vi "Raw data processing-Ref frame data.vi"(9 "Frame Data in":T5, 11 "Logging queue element":T1={"Imaging Protocol"=enum."Live Imaging", "Number of Trials"=0, "Frame Size"=512, "# Averaged frames"=0, "Dwell time (us)"=0.0, "Index of Z-plane"=0, "Timelapse?"=FALSE, "Logging process is active"=FALSE, "Speed logging enabled"=FALSE, "tdms file ref"=refnum, "path"=path "", "Trial Number"=0, "Expected # points acquired"=FALSE, "Manually stopped"=FALSE, "Last trial"=FALSE, "Ch0 data"=[], "Ch1 data"=[], "Ref Data"=[], "Ref Frame Time"=[], "Image Time"=[], "Continuous Time"=[], "Ref X Length"=0, "Ref Y Length"=0, "# Ref Averaged frames"=0, "Ref Dwell time (us)"=0.0, "Points acquired"={"Ch0 last trial"=0, "Ch1 last trial"=0, "All trials"=0}, "HW Timings File"=refnum} {"Ref Dwell time (us)" format="%#.6g"; "Frame Size" items=["100X100"=100, "128X128"=128, "200X200"=200, "256X256"=256, "512X512"=512, "1024x1024"=1024, "2048x2048"=2048]; "Dwell time (us)" format="%#.6g"}) -> (1 "Frame Data":T5, 2 "Number of points in completed Ref frame":i32, 3 "Ref Frame completed/generate image":bool, 5 "Movement Correction":bool)   [LabVIEW 2017]
uses:
  Typedefs/Frame data dual cluster.ctl
  Typedefs/Logging queue element.ctl
  Typedefs/Imaging Protocols enum.ctl
  Typedefs/Frame Size.ctl
  Typedefs/Acquired points count.ctl
  Global Variables/General Globals.vi
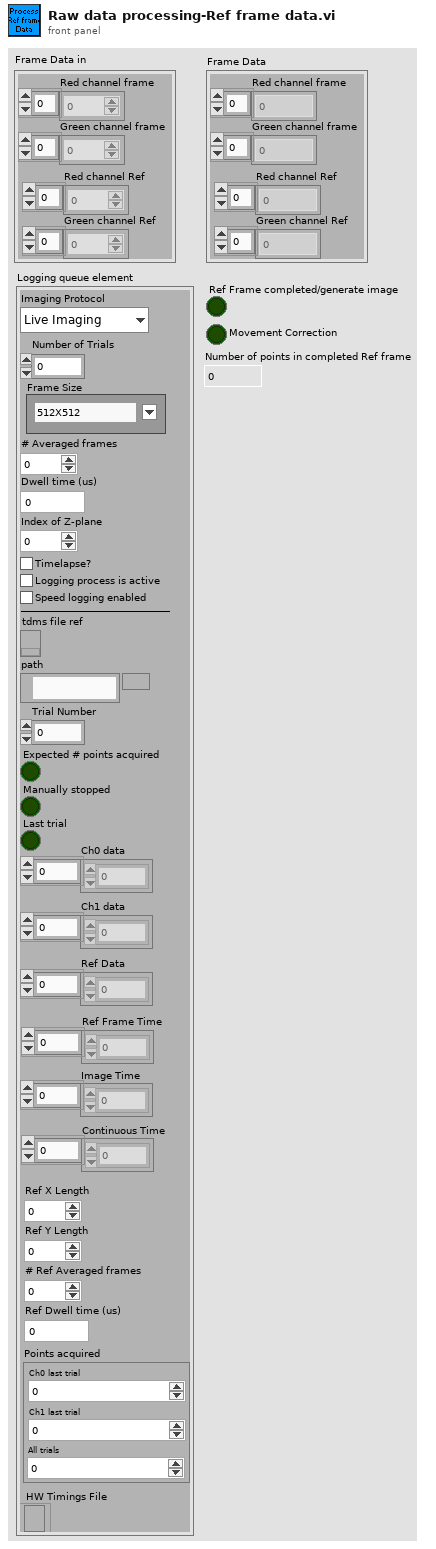
[diagram p1: front panel]
types:
  T1 = typedef "Logging queue element.ctl" = cluster{"Imaging Protocol":T2, "Number of Trials":u16, "Frame Size":T3, "# Averaged frames":u16, "Dwell time (us)":dbl, "Index of Z-plane":i32, "Timelapse?":bool, "Logging process is active":bool, "Speed logging enabled":bool, "tdms file ref":refnum<k34>, "path":path, "Trial Number":i32, "Expected # points acquired":bool, "Manually stopped":bool, "Last trial":bool, "Ch0 data":u32[], "Ch1 data":u32[], "Ref Data":u32[], "Ref Frame Time":u64[], "Image Time":u64[], "Continuous Time":u64[], "Ref X Length":u16, "Ref Y Length":u16, "# Ref Averaged frames":u16, "Ref Dwell time (us)":dbl, "Points acquired":T4, "HW Timings File":refnum<file>}
  T2 = typedef "Imaging Protocols enum.ctl" = enum16{"AOL Z-Stack", "Motor Z Stack", "Functional Acquisition", "Single Plane Acquisition", "Volume Acquisition", "Live Imaging", "Live Plane Imaging", "Live Volume Imaging"}
  T3 = typedef "Frame Size.ctl" = u16
  T4 = typedef "Acquired points count.ctl" = cluster{"Ch0 last trial":u64, "Ch1 last trial":u64, "All trials":u64}
  T5 = typedef "Frame data dual cluster.ctl" = cluster{"Red channel frame":dbl[], "Green channel frame":dbl[], "Red channel Ref":dbl[], "Green channel Ref":dbl[]}
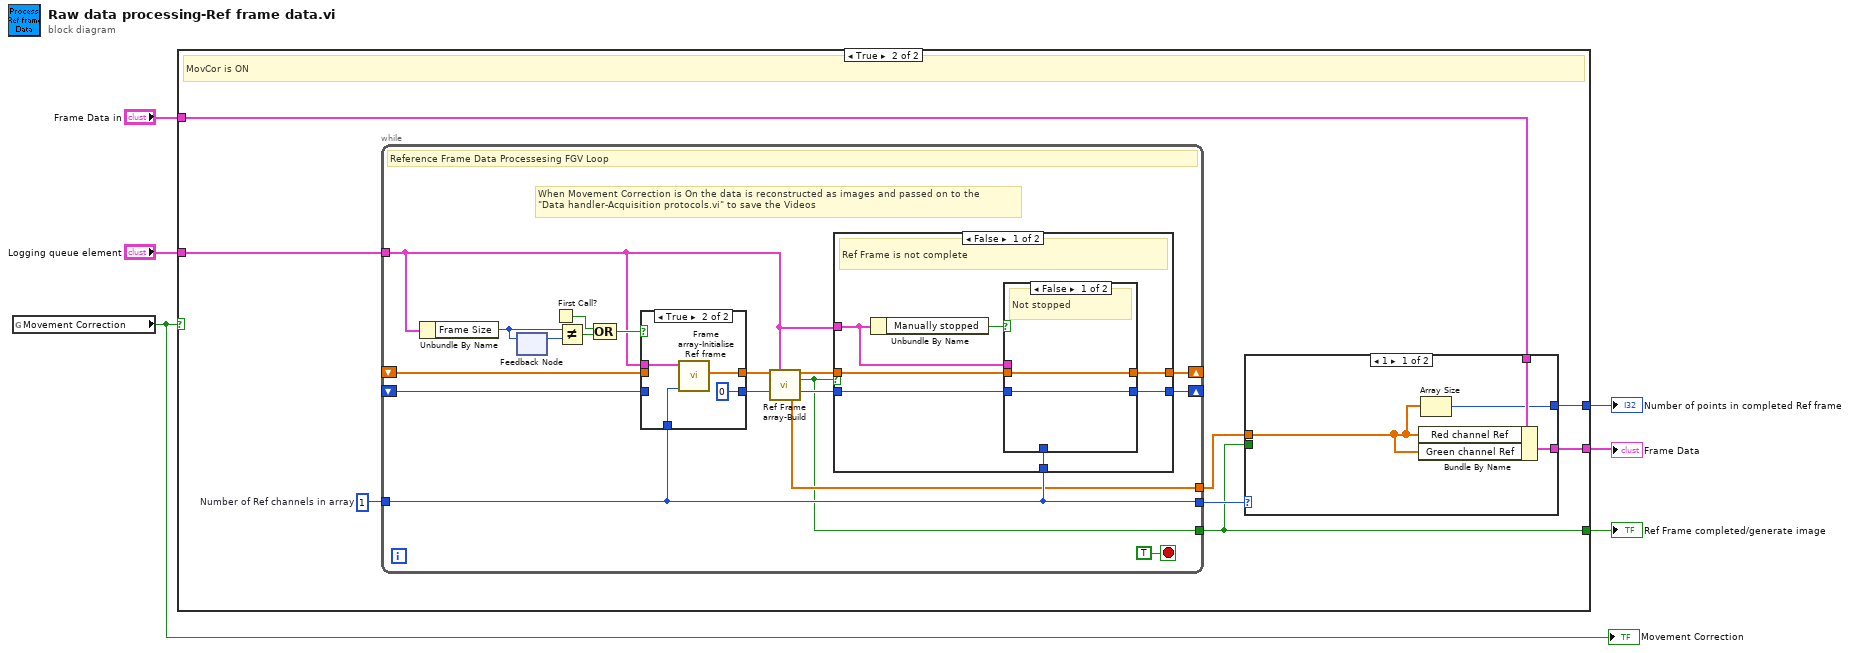
[diagram p0: block diagram]
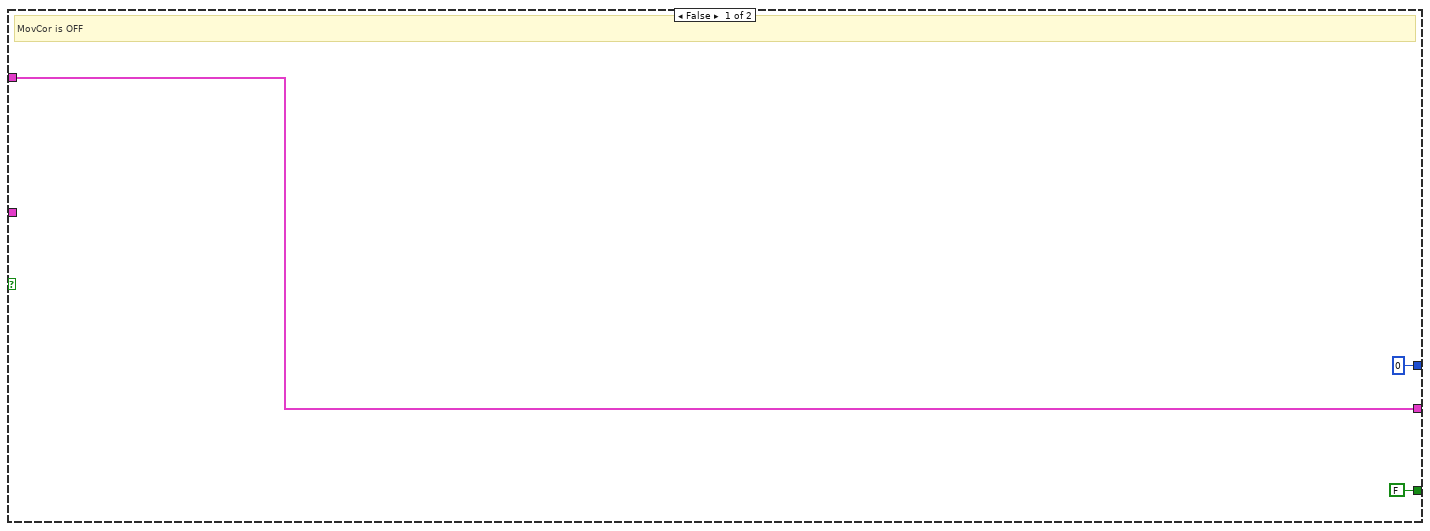
[diagram p2: hidden frame]
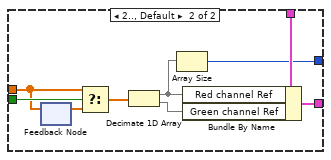
[diagram p3: hidden frame]
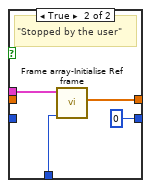
[diagram p4: hidden frame]
diagram:
  n1 = global read "General Globals.vi" "Movement Correction"() -> (w1:bool)
  "Movement Correction" <- w1
  n2 = case shown="True" w1 {
    tunnel: "Frame Data in" -> [w9 w16]
    tunnel: [w9 w15] -> w5
    tunnel: "Logging queue element" -> [_ w14]
    tunnel: [FALSE ("Ref frame completed/generate image") w11] -> w3
    tunnel: [0 w10] -> w2
    frame False {
      # "MovCor is OFF"
    }
    frame True {
      w17 = 1  # Number of Ref channels in array
      # "MovCor is ON"
      n3 = while {
        tunnel: w14 -> [w31]
        shift-right: [w36] -> _
        shift-left: _ -> [w43]
        shift-right: [w35] -> _
        shift-left: _ -> [w42]
        tunnel: [w33] -> w12
        tunnel: [w37] -> w13
        tunnel: w17 -> [w37]
        tunnel: [w32] -> w11
        stop <- TRUE stop-if-true
        # "When Movement Correction is On the data is reconstructed as images and passed on to the\n\"Data handler-Acquisition protocols.vi\" to save the Videos"
        # "Reference Frame Data Processesing FGV Loop"
        n4 = Unbundle By Name(w31) -> ("Frame Size"=w44:T3)
        n5 = feedback #1() -> (w45:T3)  [unwired: 1 in]
        n6 = feedback-in #1(w44) -> ()
        n7 = First Call?() -> (First Call?: T/F=w47:bool)
        n8 = Not Equal?(x=w44, y=w45) -> (x != y?=w46:bool)
        n9 = Compound Arithmetic op=OR(w47, w46) -> (w41:bool)
        n10 = case shown="True" w41 {
          tunnel: [w65 w66] -> w40
          tunnel: w43 -> [w65 _]
          tunnel: w31 -> [_ w69]
          tunnel: w42 -> [w64 _]
          tunnel: [w64 0 ("Count")] -> w34
          tunnel: w37 -> [_ w67]
          frame False {
          }
          frame True {
            n11 = call "Frame array-Initialise Ref frame.vi"("Number of Ref channels in array"=w67, "Logging queue element"=w69) -> ("Ref Frame-size data array (single channel)"=w66:dbl[])  [unwired: 9 in]
          }
        }
        n12 = call "Ref Frame array-Build.vi"("Single-frame buffer (in)"=w40, "Logging queue element"=w31, "Number of points in single Ref frame buffer (in)"=w34) -> ("Ref Frame Data"=w33:dbl[], "Single Ref frame buffer (out)"=w38:dbl[], "Ref frame completed/generate image"=w32:bool, "Number of points in single Ref frame buffer"=w39:i32)  [unwired: 9 in]
        n13 = case shown="False" w32 {
          tunnel: w38 -> [w53 w63]
          tunnel: [w55 w63] -> w36
          tunnel: w39 -> [w51 w62]
          tunnel: [w50 w62] -> w35
          tunnel: w31 -> [w52 _]
          tunnel: w37 -> [w49 _]
          frame False {
            # "Ref Frame is not complete"
            n14 = Unbundle By Name(w52) -> ("Manually stopped"=w54:bool)
            n15 = case shown="False" w54 {
              tunnel: [w57 w58] -> w55
              tunnel: w53 -> [w57 _]
              tunnel: w52 -> [_ w61]
              tunnel: w51 -> [w56 _]
              tunnel: [w56 0 ("Count")] -> w50
              tunnel: w49 -> [_ w59]
              frame False {
                # "Not stopped"
              }
              frame True {
                # "\"Stopped by the user\""
                n16 = call "Frame array-Initialise Ref frame.vi"("Number of Ref channels in array"=w59, "Logging queue element"=w61) -> ("Ref Frame-size data array (single channel)"=w58:dbl[])  [unwired: 9 in]
              }
            }
          }
          frame True {
            # "Ref Frame completed"
          }
        }
      }
      n17 = case shown="1" w13 {
        tunnel: [w21 w29] -> w15
        tunnel: w16 -> [w20 w28]
        tunnel: w11 -> [_ w25]
        tunnel: w12 -> [w19 w24]
        tunnel: [w18 w22] -> w10
        frame 1 {
          n18 = Bundle By Name(cluster=w20, "Red channel Ref"=w19, "Green channel Ref"=w19) -> (w21:T5)
          n19 = Array Size(array=w19) -> (size(s)=w18:i32)
        }
        frame 2.., Default {
          n20 = feedback #2() -> (w27:dbl[])  [unwired: 1 in]
          n21 = feedback-in #2(w24) -> ()
          n22 = Select(t=w24, s=w25, f=w27) -> (s? t:f=w26:dbl[])
          n23 = Decimate 1D Array(w26) -> (w23:dbl[], w30:dbl[])
          n24 = Array Size(array=w23) -> (size(s)=w22:i32)
          n25 = Bundle By Name(cluster=w28, "Red channel Ref"=w23, "Green channel Ref"=w30) -> (w29:T5)
        }
      }
    }
  }
  "Frame Data" <- w5
  "Ref Frame completed/generate image" <- w3
  "Number of points in completed Ref frame" <- w2
